vi "duplicate.vi"(8 "error in":errorcluster, 11 "configuration in":refnum<class "NISE_CEF_serializable configuration.lvclass">) -> (0 "error out":errorcluster, 2 "duplicate configuration out":refnum<class "NISE_CEF_serializable configuration.lvclass">, 3 "original configuration out":refnum<class "NISE_CEF_serializable configuration.lvclass">)   [LabVIEW 2013, in "NISE_CEF_serializable configuration.lvclass"]
uses:
  NISE_CEF_serializable configuration.lvclass
  NISE_CEF_serializable configuration.lvclass/NISE_CEF_serializable configuration.ctl
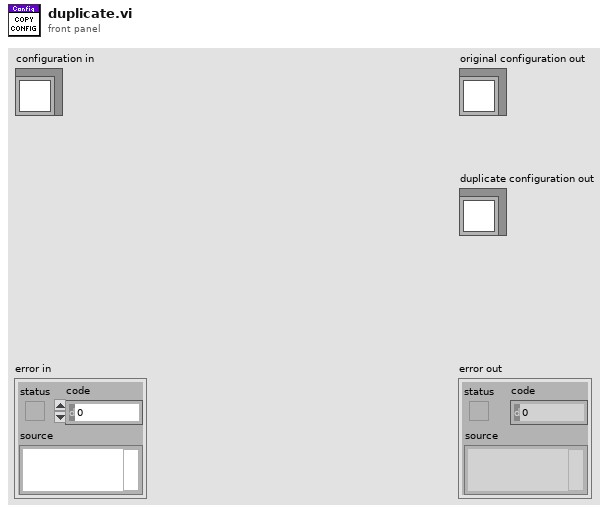
[diagram p1: front panel]
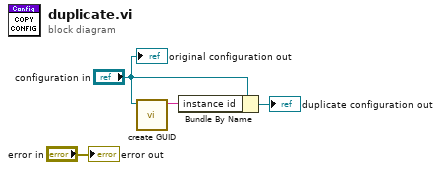
[diagram p0: block diagram]
diagram:
  n1 = call-dynamic "create GUID.vi"("configuration"="configuration in") -> ("uuid"=w3:string)  [unwired: 10 in]
  n2 = Bundle By Name(cluster="configuration in", "instance id"=w3) -> (→"duplicate configuration out":refnum<class "NISE_CEF_serializable configuration.lvclass">)
  "error out" <- "error in"
  "original configuration out" <- "configuration in"
